vi "autonomous main.vi"() -> ()   [LabVIEW 2011]
panel:
  out "Numeric 2":i32
  out "Numeric":i32
  in  "error in (no error)":errorcluster
  out "commands from file":string[][](array[string])
  out "Active Commands":string[][](array[string])
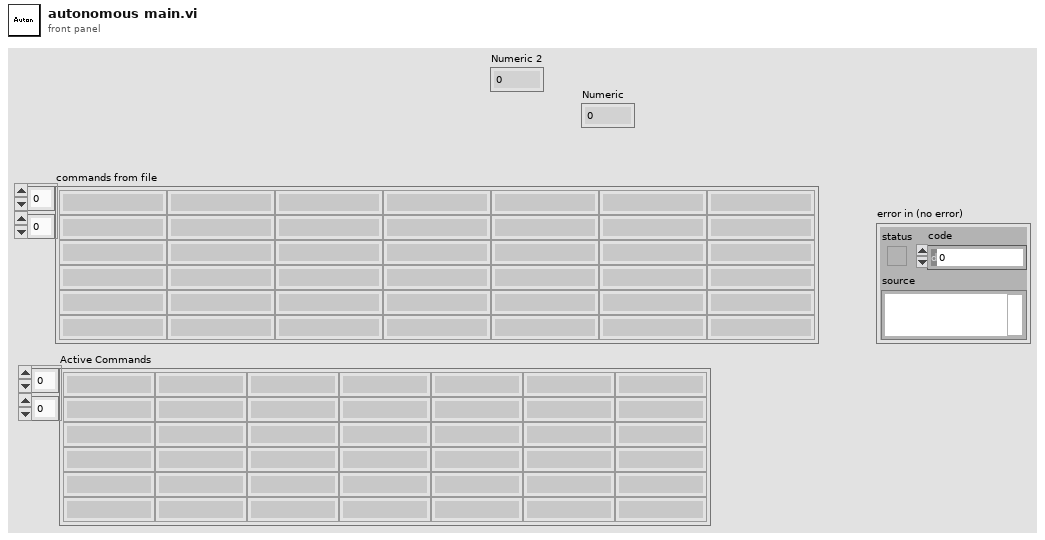
[diagram p1: front panel]
types:
  T1 = typedef "WPI_MotorControlDeviceRef.ctl" = cluster{"DeviceStatus":errorcluster, "Type":enum16{"PWM", "CAN"}, "PWM":cluster{"Digital Module":T2, "PWM Channel":T3, "DeadBand":T4}, "CAN":cluster{"Device Number":u8, "Control Mode":T5, "Semaphore":T6, "Max Vout":dbl}, "Invert":bool, "TransformRef":T7, "InvTransformRef":T7}
  T2 = typedef "FPGA_TypedefDigitalModule.ctl" = enum16{"Digital Module 1", "Digital Module 2"}
  T3 = typedef "FPGA_DIOPWMChannel.ctl" = enum8{"PWM 1", "PWM 2", "PWM 3", "PWM 4", "PWM 5", "PWM 6", "PWM 7", "PWM 8", "PWM 9", "PWM 10", "Invalid"}
  T4 = typedef "WPI_PWMDeadband.ctl" = cluster{"Name":string, "maxPositivePwm":i32, "minPositivePwm":i32, "centerPwm":i32, "maxNegativePwm":i32, "minNegativePwm":i32, "angularRange":u16}
  T5 = typedef "WPI_CANJaguar_ControlMode.ctl" = enum8{"Percent VBus", "Current", "Speed", "Position", "Voltage"}
  T6 = typedef "Semaphore RefNum" = refnum<k1>
  T7 = typedef "WPI_PWMTransform_ConPane.ctl" = refnum<vi>
  T8 = cluster{"elapsed auton time":dbl, "left encoder":dbl, "other eye":bool, "right encoder":dbl, "Angle":dbl}
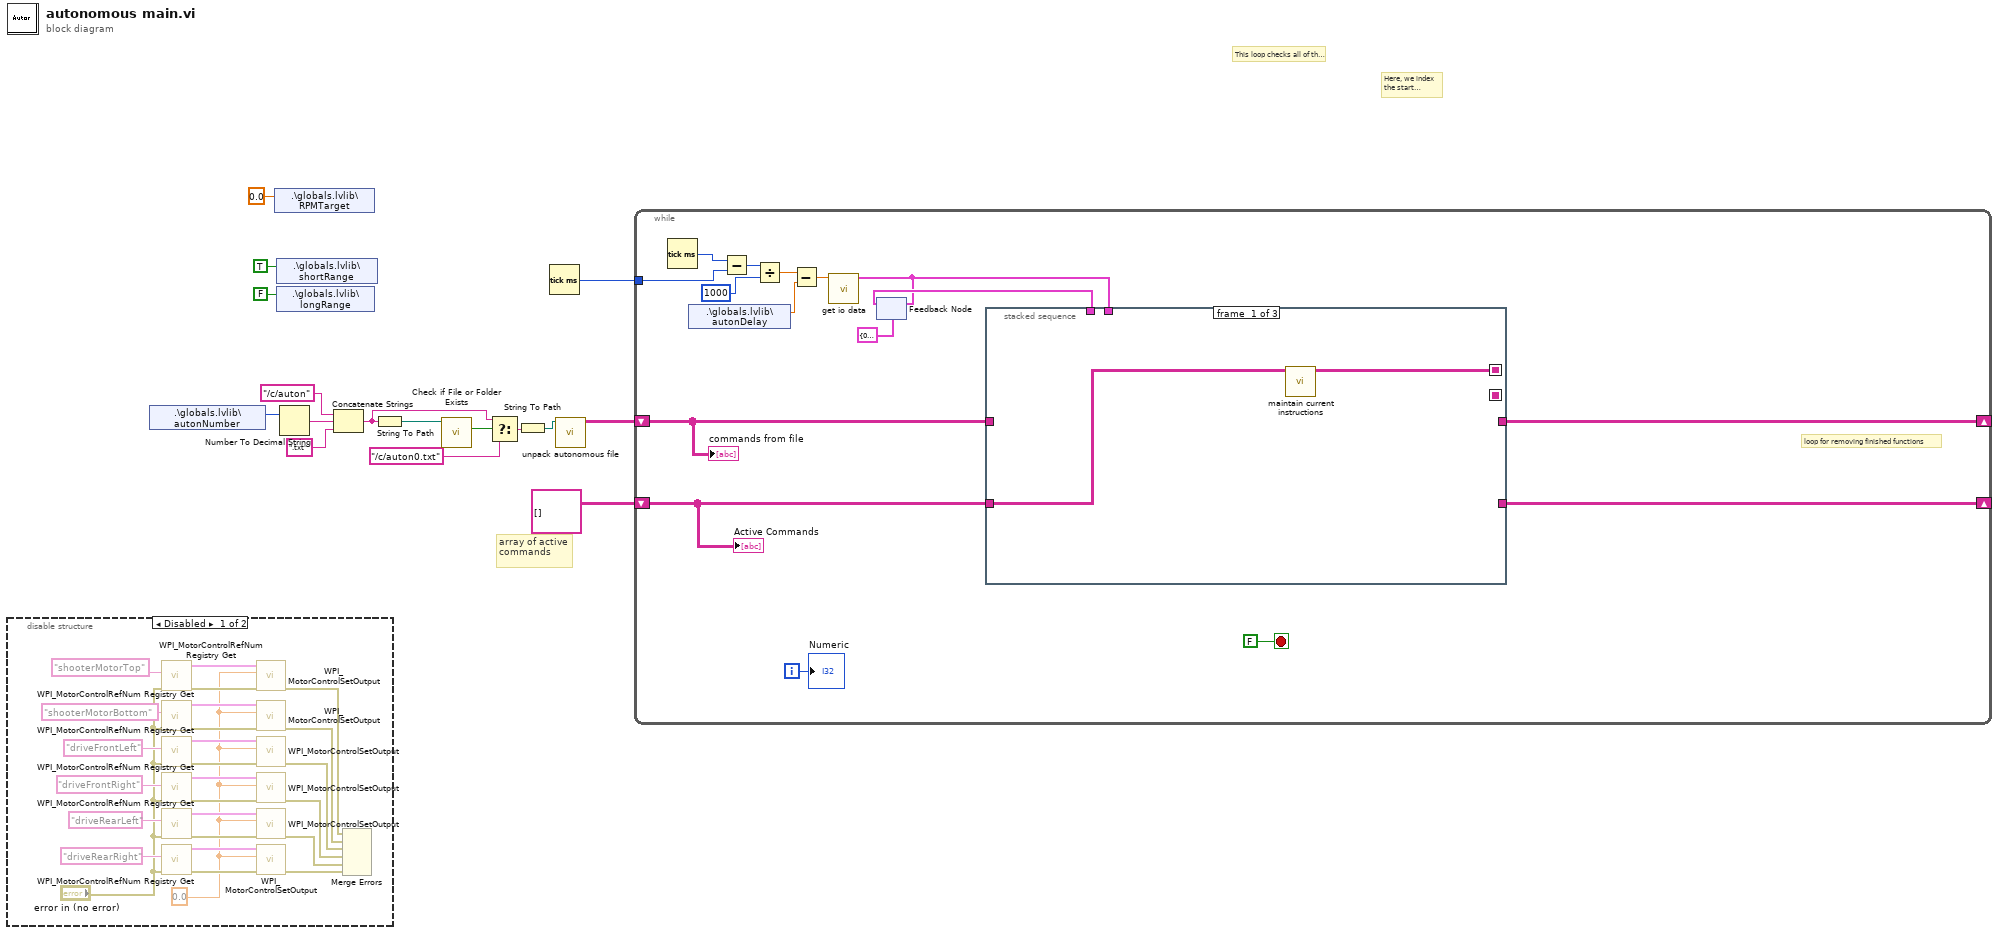
[diagram p0: block diagram]
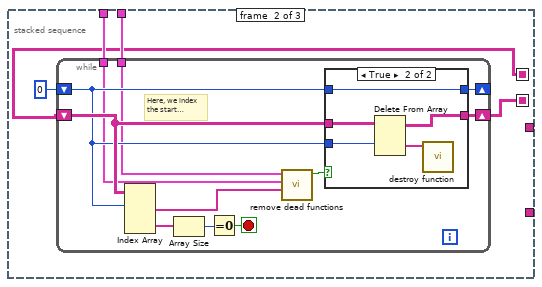
[diagram p3: hidden frame]
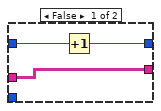
[diagram p4: hidden frame]
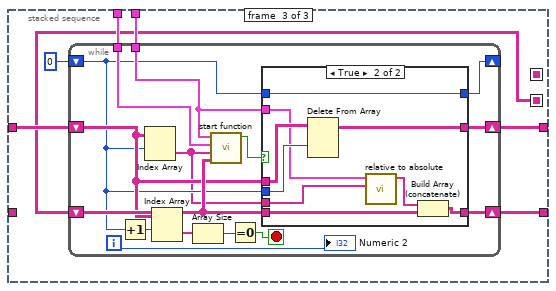
[diagram p5: hidden frame]
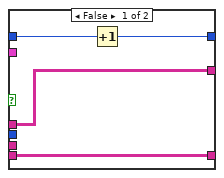
[diagram p6: hidden frame]
diagram:
  # "This loop checks all of the commands in the command/parameter array and adds the appropiate ones to the list of commands currently being executed."
  # "Here, we index the start condition type and value."
  # "array of active commands"
  n1 = disable-structure shown="Disabled" {
    frame Disabled {
      w24 = 0.0 ("Output")
      n2 = call <vilib>:"WPI_MotorControlRefNum Registry Get.vi"("error in (no error)"="error in (no error)", "refnum name"="shooterMotorTop") -> ("error out"=w38:errorcluster, "MotorControlDevRef"=w40:T1)  [unwired: 8 in]
      n3 = call <vilib>:"WPI_MotorControlRefNum Registry Get.vi"("error in (no error)"="error in (no error)", "refnum name"="shooterMotorBottom") -> ("error out"=w37:errorcluster, "MotorControlDevRef"=w39:T1)  [unwired: 8 in]
      n4 = call <vilib>:"WPI_MotorControlRefNum Registry Get.vi"("error in (no error)"="error in (no error)", "refnum name"="driveFrontLeft") -> ("error out"=w28:errorcluster, "MotorControlDevRef"=w32:T1)  [unwired: 8 in]
      n5 = call <vilib>:"WPI_MotorControlRefNum Registry Get.vi"("error in (no error)"="error in (no error)", "refnum name"="driveFrontRight") -> ("error out"=w27:errorcluster, "MotorControlDevRef"=w31:T1)  [unwired: 8 in]
      n6 = call <vilib>:"WPI_MotorControlRefNum Registry Get.vi"("error in (no error)"="error in (no error)", "refnum name"="driveRearLeft") -> ("error out"=w26:errorcluster, "MotorControlDevRef"=w30:T1)  [unwired: 8 in]
      n7 = call <vilib>:"WPI_MotorControlRefNum Registry Get.vi"("error in (no error)"="error in (no error)", "refnum name"="driveRearRight") -> ("error out"=w25:errorcluster, "MotorControlDevRef"=w29:T1)  [unwired: 8 in]
      n8 = call <vilib>:"WPI_MotorControlSetOutput.vi"("error in (no error)"=w38, "Output"=w24, "MotorControlDevRef"=w40) -> ("error out"=w22:errorcluster)  [unwired: 7 in, 1 out]
      n9 = call <vilib>:"WPI_MotorControlSetOutput.vi"("error in (no error)"=w37, "Output"=w24, "MotorControlDevRef"=w39) -> ("error out"=w21:errorcluster)  [unwired: 7 in, 1 out]
      n10 = call <vilib>:"WPI_MotorControlSetOutput.vi"("error in (no error)"=w28, "Output"=w24, "MotorControlDevRef"=w32) -> ("error out"=w20:errorcluster)  [unwired: 7 in, 1 out]
      n11 = call <vilib>:"WPI_MotorControlSetOutput.vi"("error in (no error)"=w27, "Output"=w24, "MotorControlDevRef"=w31) -> ("error out"=w19:errorcluster)  [unwired: 7 in, 1 out]
      n12 = call <vilib>:"WPI_MotorControlSetOutput.vi"("error in (no error)"=w26, "Output"=w24, "MotorControlDevRef"=w30) -> ("error out"=w18:errorcluster)  [unwired: 7 in, 1 out]
      n13 = call <vilib>:"WPI_MotorControlSetOutput.vi"("error in (no error)"=w25, "Output"=w24, "MotorControlDevRef"=w29) -> ("error out"=w17:errorcluster)  [unwired: 7 in, 1 out]
      n14 = Merge Errors(w22, w21, w20, w19, w18, w17) -> ()  [unwired: 1 out]
    }
    frame Enabled {
    }
  }
  n15 = shared-variable ".\\globals.lvlib\\autonNumber"() -> (w10:i8)  [unwired: 1 in, 1 out]
  n16 = shared-variable ".\\globals.lvlib\\RPMTarget"(0.0 ("Angle")) -> ()  [unwired: 1 in, 1 out]
  n17 = shared-variable ".\\globals.lvlib\\shortRange"(TRUE ("shortRange")) -> ()  [unwired: 1 in, 1 out]
  n18 = shared-variable ".\\globals.lvlib\\longRange"(FALSE ("longRange")) -> ()  [unwired: 1 in, 1 out]
  n19 = Number To Decimal String(number=w10) -> (decimal integer string=w8:string)  [unwired: 1 in]
  n20 = Concatenate Strings("/c/auton", w8, ".txt" ("string")) -> (w4:string)
  n21 = String To Path(string=w4) -> (path=w6:path)
  n22 = call <vilib>:"Check if File or Folder Exists.vi"("path"=w6) -> ("file or folder exists?"=w5:bool)  [unwired: 8 in, 2 out]
  n23 = Select(t=w4, s=w5, f="/c/auton0.txt") -> (s? t:f=w2:string)
  n24 = String To Path(string=w2) -> (path=w1:path)
  n25 = Tick Count (ms)() -> (millisecond timer value=w11:u32)
  n26 = call "unpack autonomous file.vi"("file path in"=w1) -> ("command/parameter array out"=w15:string[][])  [unwired: 10 in]
  n27 = while {
    shift-right: [w45] -> _
    shift-left: string[][] [] -> [w58]
    shift-right: [w46] -> _
    shift-left: w15 -> [w57]
    tunnel: w11 -> [w54]
    i -> [w55]
    stop <- FALSE stop-if-true
    # "loop for removing finished functions"
    n28 = Tick Count (ms)() -> (millisecond timer value=w50:u32)
    n29 = shared-variable ".\\globals.lvlib\\autonDelay"() -> (w47:dbl)  [unwired: 1 in, 1 out]
    n30 = Subtract(x=w50, y=w54) -> (x-y=w53:u32)
    n31 = Divide(x=w53, y=u32 1000) -> (x/y=w48:dbl)
    n32 = Subtract(x=w48, y=w47) -> (x-y=w49:dbl)
    n33 = call "get io data.vi"("elapsed auton time"=w49) -> ("sensor datas"=w43:T8)  [unwired: 10 in]
    n34 = feedback #1(T8 {"elapsed auton time"=0.0, "left encoder"=0.0, "other eye"=FALSE, "right encoder"=0.0, "Angle"=0.0} ("const")) -> (w51:T8)
    n35 = feedback-in #1(w43) -> ()
    n36 = stacked-sequence {
      seq-local: [_ w62 _] -> [_ _ w85]
      seq-local: [w60 _ _] -> [_ w61 _]
      tunnel: w58 -> [w59 _ _]
      tunnel: w57 -> [_ _ w88]
      tunnel: w43 -> [_ w63 w91]
      tunnel: w51 -> [_ w64 w90]
      tunnel: [_ _ w87] -> w46
      tunnel: [_ _ w86] -> w45
      frame #0 {
        n37 = call "maintain current instructions.vi"("running commands"=w59) -> ("running commands out"=w60:string[][])  [unwired: 7 in, 1 out]
      }
      frame #1 {
        n38 = while {
          shift-right: [w75] -> w62
          shift-left: w61 -> [w76]
          shift-right: [w73] -> _
          shift-left: 0 -> [w72]
          tunnel: w64 -> [w67]
          tunnel: w63 -> [w66]
          stop <- w69 stop-if-true
          # "Here, we index the start condition type and value."
          n39 = Index Array(array=w76, index (row) #1=w72) -> (element #1=w68:string[], element #2=w71:string[])  [unwired: 3 in]
          n40 = Array Size(array=w71) -> (size(s)=w70:i32)
          n41 = Equal To 0?(x=w70) -> (x = 0?=w69:bool)
          n42 = call "remove dead functions.vi"("command in"=w68, "old sensor datas"=w67, "sensor datas"=w66) -> ("remove"=w74:bool)  [unwired: 8 in]
          n43 = case shown="True" w74 {
            tunnel: [w79 w83] -> w75
            tunnel: w76 -> [w79 w84]
            tunnel: w72 -> [_ w82]
            tunnel: w72 -> [w78 w80]
            tunnel: [w77 w80] -> w73
            frame False {
              n44 = Increment(x=w78) -> (x+1=w77:i32)
            }
            frame True {
              n45 = Delete From Array(array=w84, index (row)=w82) -> (deleted portion=w81:string[], array with subset deleted=w83:string[][])  [unwired: 2 in]
              n46 = call "destroy function.vi"("command in"=w81) -> ()  [unwired: 11 in]
            }
          }
        }
      }
      frame #2 {
        n47 = while {
          shift-right: [w105] -> w86
          shift-left: w85 -> [w103]
          shift-right: [w104] -> w87
          shift-left: w88 -> [w99]
          tunnel: w91 -> [w101]
          tunnel: w90 -> [w102]
          shift-right: [w95] -> _
          shift-left: 0 -> [w94]
          i -> [w93]
          stop <- w96 stop-if-true
          n48 = Increment(x=w94) -> (x+1=w100:i32)
          n49 = Index Array(array=w99, index (row)=w94) -> (element=w92:string[])  [unwired: 1 in]
          n50 = Index Array(array=w99, index (row)=w100) -> (element=w98:string[])  [unwired: 1 in]
          n51 = Array Size(array=w98) -> (size(s)=w97:i32)
          n52 = call "start function.vi"("running command array"=w103, "command in"=w92, "old sensor datas"=w102, "sensor datas"=w101) -> ("start?"=w106:bool)  [unwired: 7 in]
          n53 = Equal To 0?(x=w97) -> (x = 0?=w96:bool)
          n54 = case shown="True" w106 {
            tunnel: [w110 w116] -> w104
            tunnel: w103 -> [w109 w117]
            tunnel: w92 -> [_ w114]
            tunnel: w99 -> [w110 w119]
            tunnel: w94 -> [_ w118]
            tunnel: [w109 w115] -> w105
            tunnel: w101 -> [_ w113]
            tunnel: [w107 w112] -> w95
            tunnel: w94 -> [w108 w112]
            frame False {
              n55 = Increment(x=w108) -> (x+1=w107:i32)
            }
            frame True {
              n56 = Delete From Array(array=w119, index (row)=w118) -> (array with subset deleted=w116:string[][])  [unwired: 2 in, 1 out]
              n57 = call "relative to absolute.vi"("command in"=w114, "datas"=w113) -> ("adjusted command"=w111:string[])  [unwired: 9 in]
              n58 = Build Array (concatenate)(w111, w117) -> (w115:string[][])
            }
          }
          "Numeric 2" <- w93
        }
      }
    }
    "Active Commands" <- w58
    "commands from file" <- w57
    "Numeric" <- w55
  }
